vi "FGV Central Message Logger.vi"(7 "Write? (F)":bool, 8 "Error In":errorcluster, 11 "CS++MessageLogger in":refnum<class "CS++MessageLogger.lvclass">) -> (0 "Error Out":errorcluster, 3 "CS++MessageLogger out":refnum<class "CS++MessageLogger.lvclass">)   [LabVIEW 2016, in "CS++Base.lvlib"]
doc: "This is a FGV storing the central CS++MessageLogger object."
uses:
  CS++Base.lvlib
  Classes/CS++BaseClasses/MessageLogger/CS++MessageLogger.lvclass
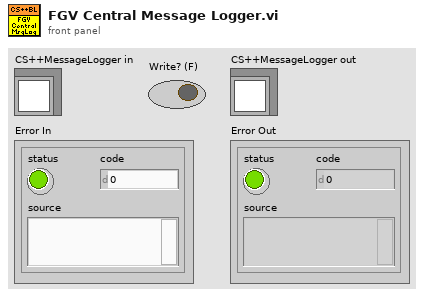
[diagram p1: front panel]
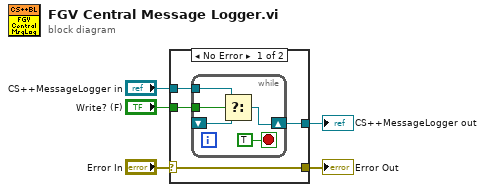
[diagram p0: block diagram]
diagram:
  n1 = case shown="No Error" "Error In" {
    selector: "Error In" -> [w6 _]
    tunnel: "CS++MessageLogger in" -> [w9 w15]
    tunnel: "Write? (F)" -> [w8 _]
    tunnel: [w7 w15] -> w3
    tunnel: [w6 _] -> w1
    frame No Error {
      n2 = while {
        shift-right: [w11] -> w7
        shift-left: _ -> [w13]
        tunnel: w9 -> [w12]
        tunnel: w8 -> [w10]
        stop <- TRUE stop-if-true
        n3 = Select(t=w12, s=w10, f=w13) -> (s? t:f=w11:refnum<class "CS++MessageLogger.lvclass">)
      }
    }
    frame Error {
    }
  }
  "CS++MessageLogger out" <- w3
  "Error Out" <- w1
